vi "scratch.vi"() -> ()   [LabVIEW 2020]
panel:
  in  "DataPaths":T1
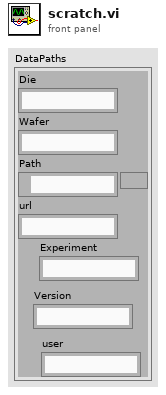
[diagram p1: front panel]
types:
  T1 = cluster{"Die":string, "Wafer":string, "Path":path, "url":string, "Experiment":string, "Version":string, "user":string}
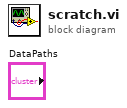
[diagram p0: block diagram]
diagram:
